vi "显示一组测试结果.vi"(4 "量测项名称":string[](array[string]), 6 "是否显示结果":bool[](array[boolean]), 8 "显示坐标":cluster{dbl, "Numeric":dbl}[](array[cluster])=[{300.0, "Numeric"=200.0}, {300.0, "Numeric"=400.0}, {300.0, "Numeric"=600.0}], 9 "单个结果":bool[](array[boolean]), 10 "待写入数据":dbl[](array[numeric]), 11 "Img":T1) -> ()   [LabVIEW 2014]
uses:
  <vilib>/vision/Image Controls.llb/IMAQ Image.ctl
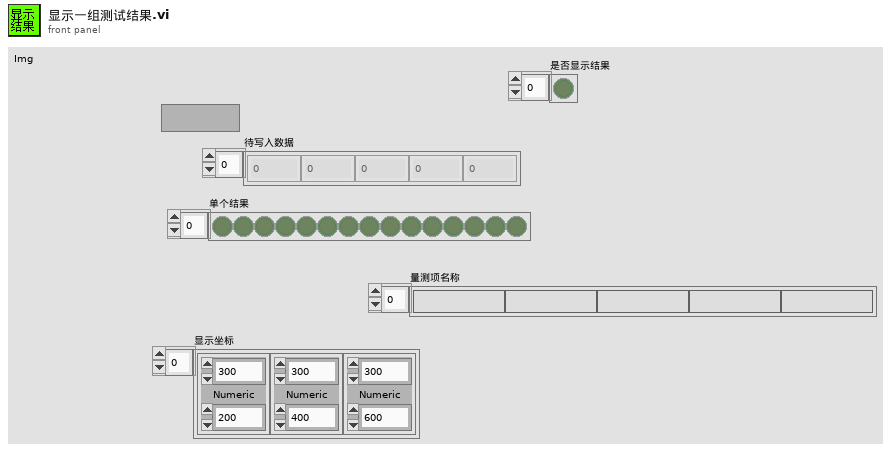
[diagram p1: front panel]
types:
  T1 = typedef "IMAQ Image.ctl" = refnum<image>
  T2 = cluster{"Desired Font (Application)":enum16{"User-specified Font", "Application Font", "System Font", "Dialog Font"}, "[User-specified Font]":cluster{"Font Name":string, "Size":i16, "Strikeout?":bool, "Italic?":bool, "Underline?":bool, "Outline?":bool, "Shadow?":bool, "Bold?":bool, "Rotation Angle":dbl}, "Horizontal Alignment":i16, "Vertical Alignment":i16}
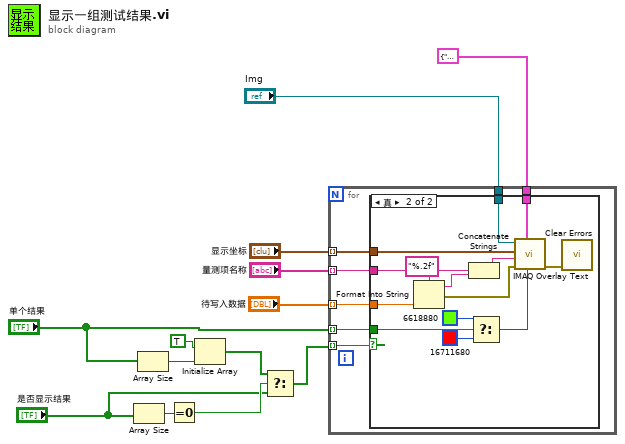
[diagram p0: block diagram]
diagram:
  n1 = Array Size(array="是否显示结果") -> (size(s)=w11:i32)
  n2 = Array Size(array="单个结果") -> (size(s)=w10:i32)
  n3 = Equal To 0?(x=w11) -> (x = 0?=w8:bool)
  n4 = Initialize Array(TRUE, w10) -> (w7:bool[])
  n5 = Select(t=w7, s=w8, f="是否显示结果") -> (s? t:f=w5:bool[])
  n6 = for {
    tunnel: "Img" -> [w20]
    tunnel: "待写入数据" -> [w19] mode=indexing
    tunnel: "显示坐标" -> [w17] mode=indexing
    tunnel: "单个结果" -> [w18] mode=indexing
    tunnel: w5 -> [w16] mode=indexing
    tunnel: T2 {"Desired Font (Application)"=enum."User-specified Font", "[User-specified Font]"={"Font Name"="", "Size"=120, "Strikeout?"=FALSE, "Italic?"=FALSE, "Underline?"=FALSE, "Outline?"=FALSE, "Shadow?"=FALSE, "Bold?"=FALSE, "Rotation Angle"=0.0}, "Horizontal Alignment"=0, "Vertical Alignment"=0} ("Font, Size & Style") -> [w15]
    tunnel: "量测项名称" -> [w14] mode=indexing
    n7 = case shown="真" w16 {
      tunnel: w20 -> [_ w34]
      tunnel: w19 -> [_ w33]
      tunnel: w18 -> [_ w31]
      tunnel: w17 -> [_ w25]
      tunnel: w15 -> [_ w24]
      tunnel: w14 -> [_ w23]
      frame False {
      }
      frame True {
        n8 = Format Into String(format string="%.2f" ("格式字符串"), w33) -> (resulting string=w22:string, error out=w27:errorcluster)  [unwired: 2 in]
        n9 = Concatenate Strings(w23, w22) -> (w21:string)
        n10 = Select(t=u32 6618880 ("Text Color (black)"), s=w31, f=u32 16711680 ("Text Color (black)")) -> (s? t:f=w28:u32)
        n11 = call "IMAQ Overlay Text"("Text Color (black)"=w28, "Font, Size & Style"=w24, "error in (no error)"=w27, "String"=w21, "Origin"=w25, "Image"=w34) -> ("error out"=w26:errorcluster)  [unwired: 4 in, 1 out]
        n12 = call <vilib>:"Clear Errors.vi"("error in (no error)"=w26) -> ()  [unwired: 5 in, 2 out]
      }
    }
  }
